vi "Test_RW Tag.vi"() -> ()   [LabVIEW 2017]
uses:
  2aaa8611-9c87-45a3-bea6-b6dd87273457.vi
  5c73c451-cd86-420b-bccf-a57af6073fd2.vi
  2fa3edc3-5848-4cd7-9023-ce10a22e5421.vi
  36280ab7-ed75-4168-88f6-4d6be7e44e63.vi
panel:
  in  "milliseconds to wait":u32=100
  out "Numeric 2":i32=81
  out "Numeric":i32=81
  in  "stop":bool
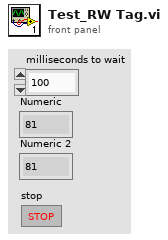
[diagram p1: front panel]
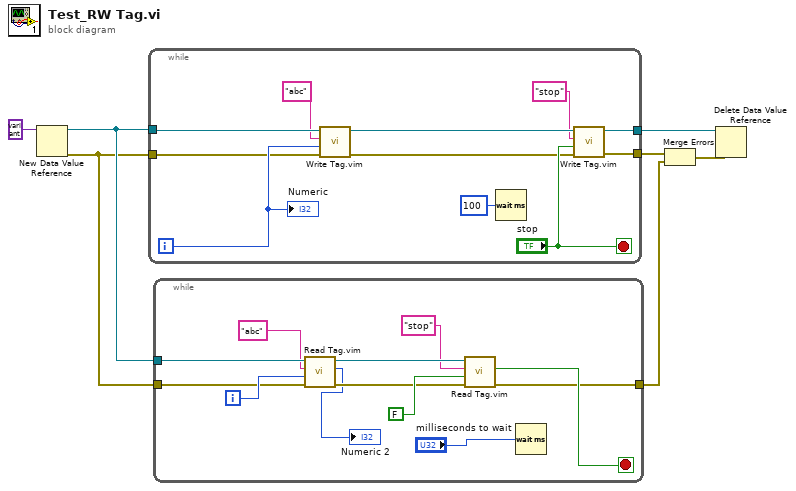
[diagram p0: block diagram]
diagram:
  n1 = New Data Value Reference(data value=variant) -> (data value reference=w6:refnum<data-value>, error out=w1:errorcluster)  [unwired: 1 in]
  n2 = while {
    tunnel: w6 -> [w18]
    tunnel: [w11] -> w5
    tunnel: [w10] -> w3
    tunnel: w1 -> [w9]
    i -> [w16]
    stop <- "stop" stop-if-true
    n3 = call "Write Tag.vim"("error in (no error)"=w9, "Value"=w16, "name"="abc", "TagMap"=w18) -> ("error out"=w8:errorcluster, "TagMap(dup)"=w14:refnum<data-value>)  [unwired: 6 in]
    n4 = Wait (ms)(milliseconds to wait=u32 100) -> ()  [unwired: 1 out]
    n5 = call "Write Tag.vim"("error in (no error)"=w8, "Value"="stop", "name"="stop", "TagMap"=w14) -> ("error out"=w10:errorcluster, "TagMap(dup)"=w11:refnum<data-value>)  [unwired: 6 in]
    "Numeric" <- w16
  }
  n6 = while {
    tunnel: w6 -> [w29]
    tunnel: [w22] -> w2
    tunnel: w1 -> [w21]
    i -> [w27]
    stop <- w23 stop-if-true
    n7 = call "Read Tag.vim"("error in (no error)"=w21, "Type"=w27, "name"="abc", "TagMap"=w29) -> ("error out"=w20:errorcluster, "Value"=→"Numeric 2":i32, "TagMap(dup)"=w26:refnum<data-value>)  [unwired: 4 in, 1 out]
    n8 = call "Read Tag.vim"("error in (no error)"=w20, "Type"=FALSE, "name"="stop", "TagMap"=w26) -> ("error out"=w22:errorcluster, "Value"=w23:bool)  [unwired: 4 in, 2 out]
    n9 = Wait (ms)(milliseconds to wait="milliseconds to wait") -> ()  [unwired: 1 out]
  }
  n10 = Merge Errors(w3, w2) -> (w4:errorcluster)
  n11 = Delete Data Value Reference(data value reference=w5, error in=w4) -> ()  [unwired: 2 out]
